vi "Acquire SN.vi"(8 "error in":errorcluster, 11 "Hardware Configuration in":T1 {"Reference Distance" format="%.3g"}) -> (0 "error out":errorcluster, 3 "Hardware Configuration out":T1 {"Reference Distance" format="%.3g"})   [LabVIEW 2018, in "Acquisition.lvlib"]
uses:
  Acquisition.lvlib
  Hardware Configuration.ctl
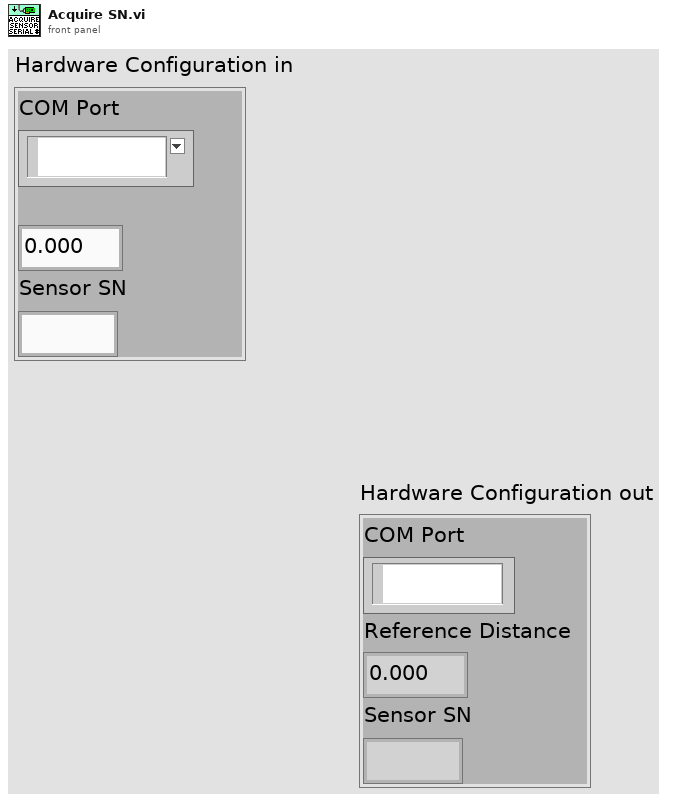
[diagram p1: front panel]
types:
  T1 = typedef "Acquisition.lvlib/Hardware Configuration.ctl" = cluster{"COM Port":refnum<visa-resource-name>, "Reference Distance":dbl, "Sensor SN":string}
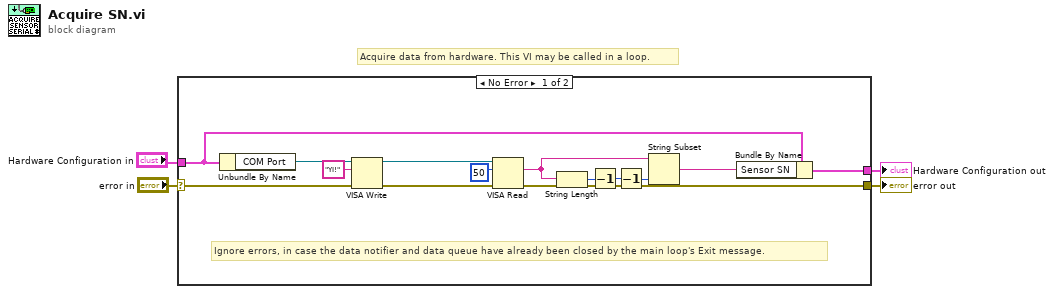
[diagram p0: block diagram]
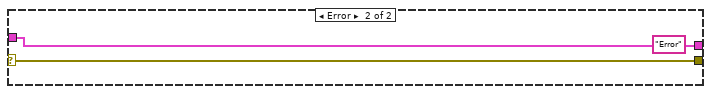
[diagram p2: hidden frame]
diagram:
  # "Acquire data from hardware. This VI may be called in a loop."
  n1 = case shown="No Error" "error in" {
    selector: "error in" -> [w17 w20]
    tunnel: [w12 w20] -> w2
    tunnel: "Hardware Configuration in" -> [w7 w19]
    tunnel: [w6 w19] -> w1
    frame No Error {
      # "Ignore errors, in case the data notifier and data queue have already been closed by the main loop's Exit message."
      n2 = Unbundle By Name(w7) -> ("COM Port"=w18:refnum<visa-resource-name>)
      n3 = VISA Write(VISA resource name=w18, write buffer="YI!", error in (no error)=w17) -> (VISA resource name out=w14:refnum<visa-resource-name>, error out=w15:errorcluster)  [unwired: 1 out]
      n4 = VISA Read(VISA resource name=w14, byte count=u32 50, error in (no error)=w15) -> (read buffer=w10:string, error out=w12:errorcluster)  [unwired: 2 out]
      n5 = String Length(string=w10) -> (length=w11:i32)
      n6 = Decrement(x=w11) -> (x-1=w9:i32)
      n7 = Decrement(x=w9) -> (x-1=w8:i32)
      n8 = String Subset(string=w10, length (rest)=w8) -> (substring=w5:string)  [unwired: 1 in]
      n9 = Bundle By Name(cluster=w7, "Sensor SN"=w5) -> (w6:T1)
    }
    frame Error {
      (unwired) "Error" ("read buffer")
    }
  }
  "error out" <- w2
  "Hardware Configuration out" <- w1
